vi "Instrument.1820.FloatApprox.vi"(1 "y":dbl, 2 "x":dbl) -> (0 "x ~ y?":bool)   [LabVIEW 2016, in "Instrument.Oxford1820.lvclass"]
doc: "Use to compare floating point numbers. This will check if two numbers are the same to 6 decimal places. Edit block diagram to change tolerance."
uses:
  Instrument.Oxford1820.lvclass
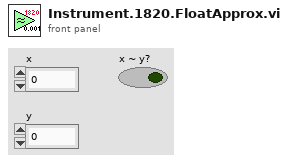
[diagram p1: front panel]
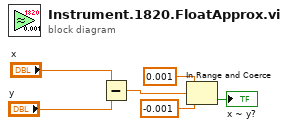
[diagram p0: block diagram]
diagram:
  n1 = Subtract(x="x", y="y") -> (x-y=w3:dbl)
  n2 = In Range and Coerce(upper limit=0.001, x=w3, lower limit=-0.001 ("upper limit")) -> (In Range?=→"x ~ y?":bool)  [unwired: 1 out]
